vi "内置参数设置.vi"() -> ()   [LabVIEW 2016]
uses:
  <vilib>/Utility/miscctls.llb/LVPointTypeDef.ctl
panel:
  in  "滴定延时时间:\n(单位:毫秒)":u16
  in  "斜率阈值:":dbl
  in  "阀配置:":u8(ring) items=["三通阀", "排阀"]
  in  "AB跨度告警值:":u16
  in  "B值告警上限值:":u16
  in  "B值范围:":u16
  in  "A值告警上限值:":u16
  in  "A值范围:":u16
  in  "是否存在液位检测板:":u16(ring) items=["否", "是"]
  in  "检出限(mg/L):":dbl
  in  "测量精度(mg/L):":dbl
  in  "ILimitDown":dbl
  in  "ILimitUp:":dbl
  in  "K d:":dbl
  in  "K i:":dbl
  in  "K p:":dbl
  in  "加热超时时间:(单位:秒)":dbl
  in  "告警温度:":dbl
  in  "加热温度:  校准参数":dbl
  in  "运行速度:  (修改需要重启)":u16
  in  "偏心轮: 校准参数":dbl
  in  "注射泵加热超时时间(s):":u16
  in  "注射泵保温温度H:":u8
  in  "注射泵\n保温温度L:":u8
  in  "废液通道:":u8
  in  "纯水通道:":u8
  in  "滴定速度:":u16
  in  "出样速度:":u16
  in  "进样速度:":u16
  in  "阀数量:":u8(ring) items=["9通"=9, "12通"=12]
  in  "注射泵型号":u8(ring) items=["TECAN", "润泽", "旋转阀"]
  in  "阈值(高→低)(mg/L):":dbl
  in  "阈值(低→高)(mg/L):":dbl
  in  "检测下限(mg/L):":dbl
  in  "检测上限(mg/L):":dbl
  in  "关闭":bool
  in  "保存":bool
  in  "读取":bool
  # "仪器内部参数设置"
  # "~"
  # "~"
  # "~"
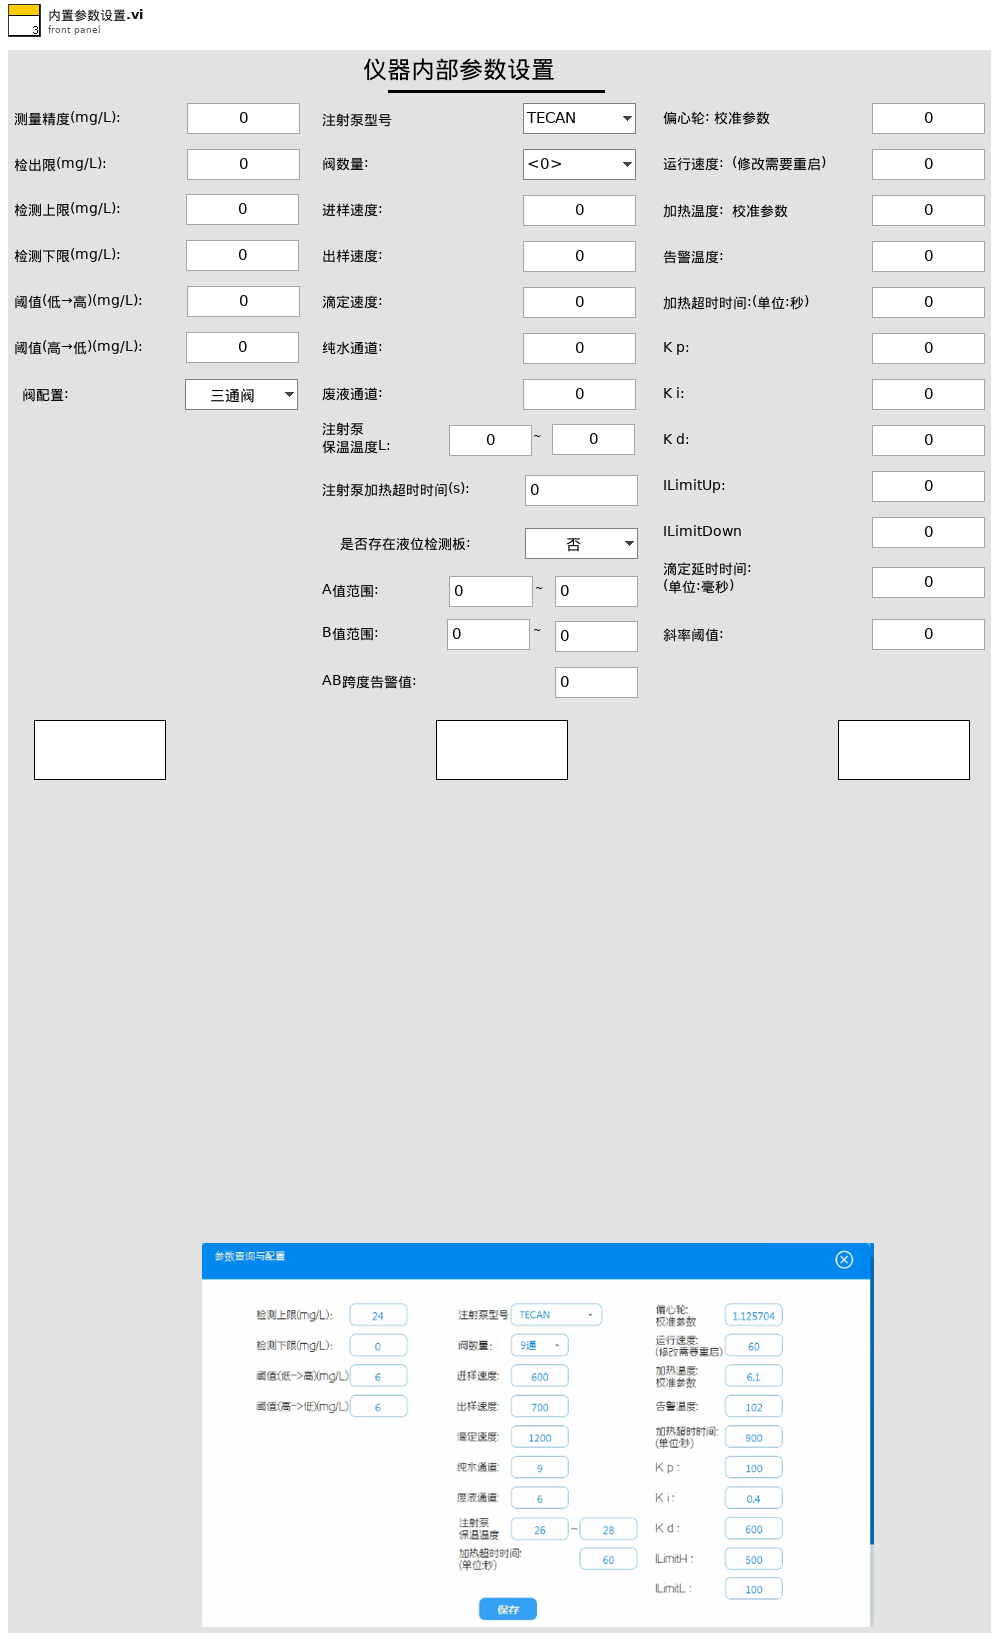
[diagram p1: front panel]
types:
  T1 = typedef "LVPointTypeDef.ctl" = cluster{"Horizontal":i16, "Vertical":i16}
  T2 = cluster{"偏心轮校准参数":dbl, "运行速度(修改需要重启)":u16, "加热温度(校准参数) ":dbl, "告警温度":dbl, "加热超时时间:(单位/秒)":dbl, "K p":dbl, "K i":dbl, "K d":dbl, "ILimitUp":dbl, "ILimitDown":dbl}
  T3 = cluster{"泵类型":u8, "阀数量":u8, "纯水通道":u8, "废液通道":u8, "进样速度":u16, "出样速度":u16, "滴定速度":u16, "注射泵保温温度L":u8, "注射泵保温温度H":u8, "注射泵加热超时时间":u16, "是否存在液位检测板":u16, "A值告警下限值":u16, "A值告警上限值":u16, "B值告警下限值":u16, "B值告警上限值":u16, "AB跨度告警值":u16, "阀配置:":u8, "滴定等待时间":u16, "滴定吸光度斜率":dbl}
  T4 = cluster{"检出限":dbl, "测量精度":dbl, "上限":dbl, "下限":dbl, "阈值（低->高）":dbl, "阈值（高->低）":dbl}
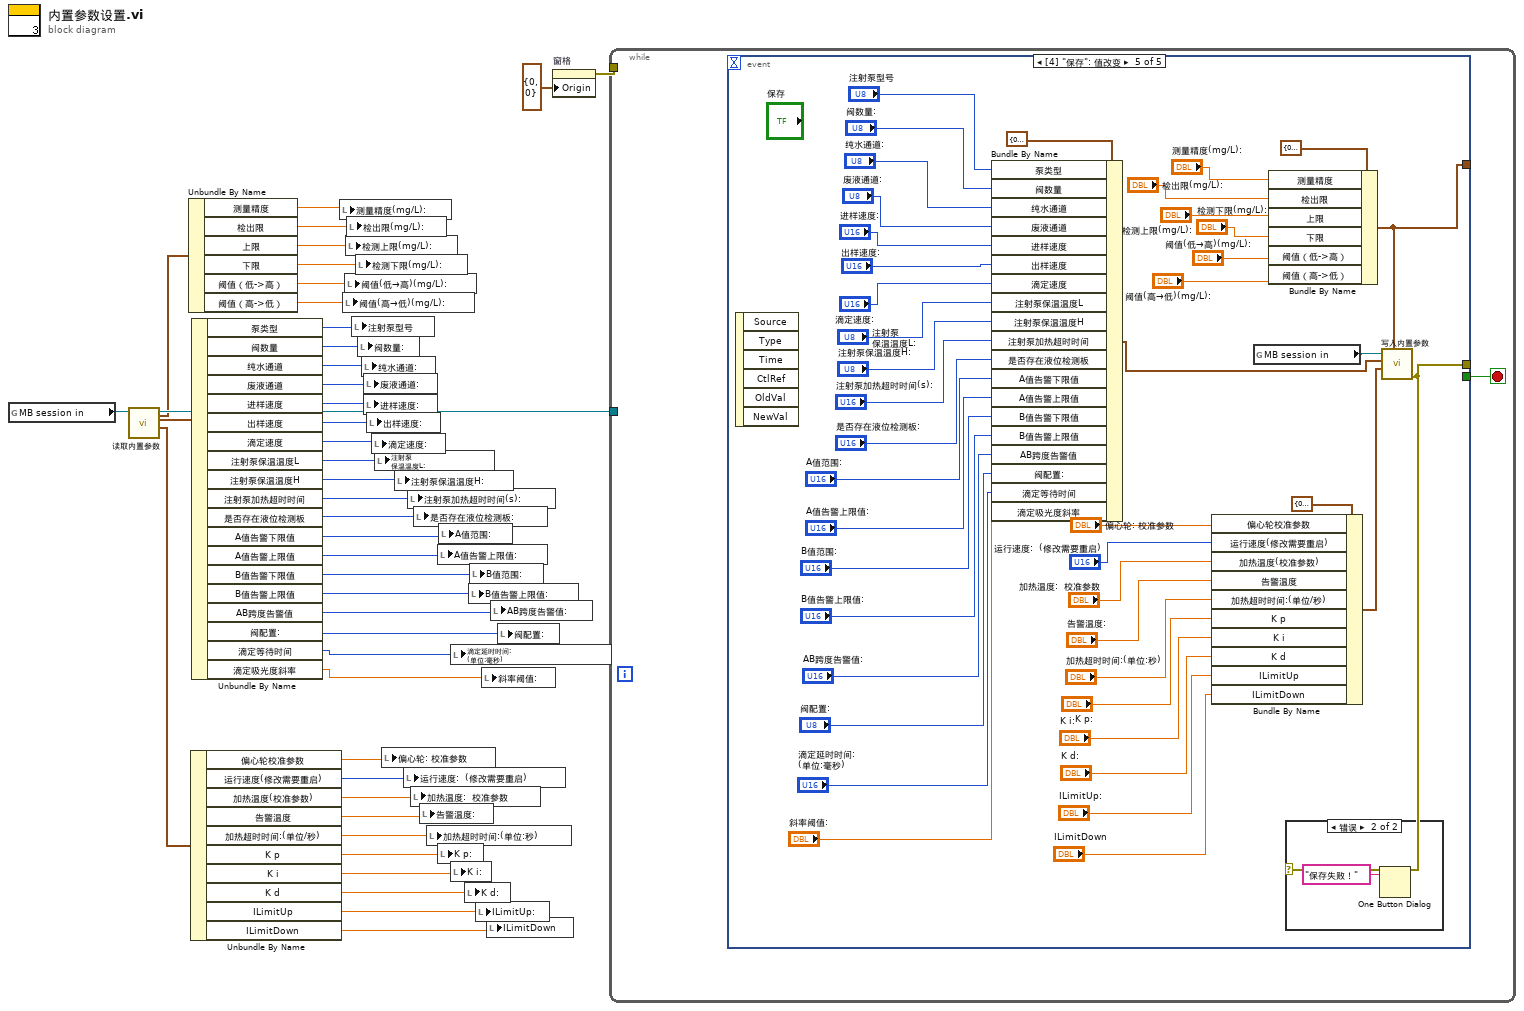
[diagram p0: block diagram]
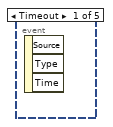
[diagram p2: hidden frame]
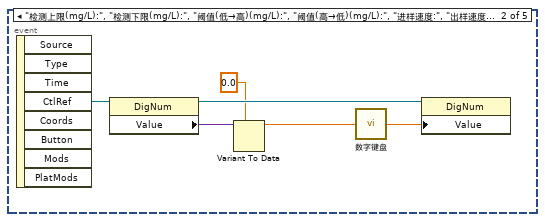
[diagram p3: hidden frame]
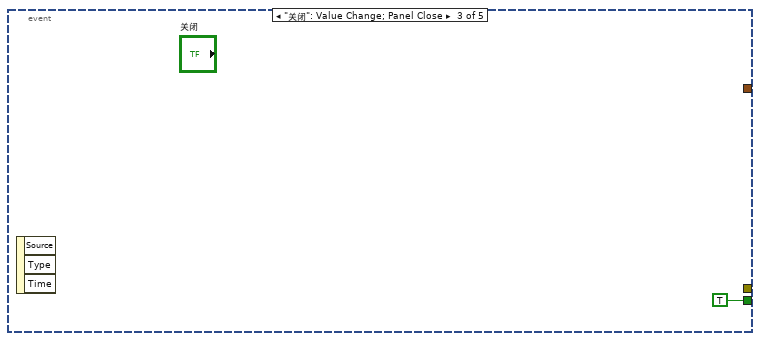
[diagram p4: hidden frame]
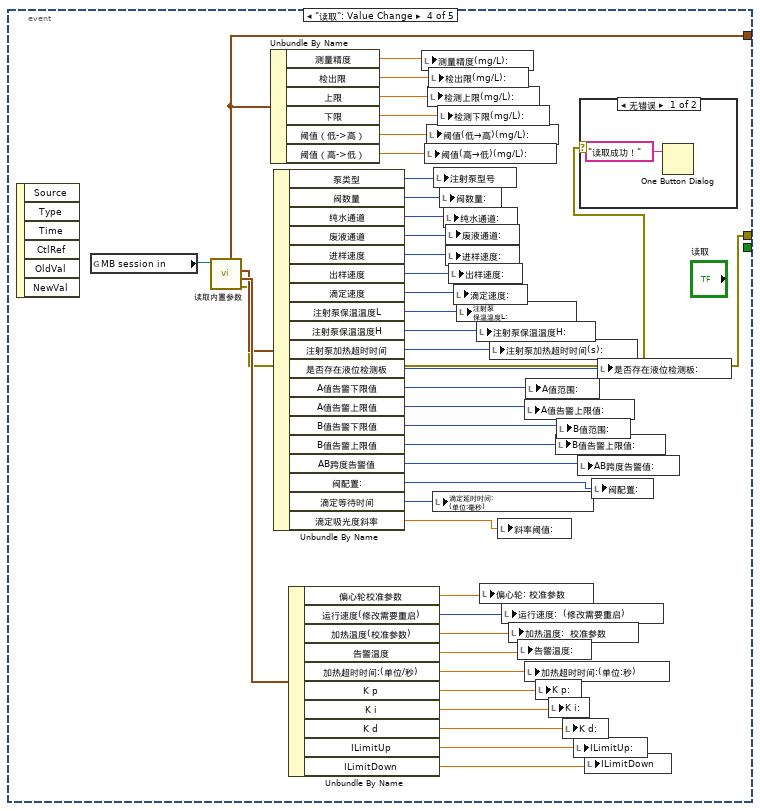
[diagram p5: hidden frame]
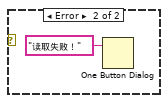
[diagram p6: hidden frame]
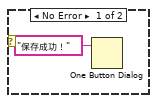
[diagram p7: hidden frame]
diagram:
  n1 = global read "VAR挥发酚全局变量.vi" "MB session in"() -> (w40:refnum<class "MB_Master.lvclass">)
  n2 = call "读取内置参数.vi"("MB session in"=w40) -> ("float"=w37:T2, "外设配置"=w38:T3, "MB session out"=w39:refnum<class "MB_Master.lvclass">, "量程参数读取"=w3:T4)  [unwired: 6 in, 1 out]
  n3 = Unbundle By Name(w3) -> ("测量精度"=w36:dbl, "检出限"=w35:dbl, "上限"=w34:dbl, "下限"=w33:dbl, "阈值（低->高）"=w32:dbl, "阈值（高->低）"=w31:dbl)
  n4 = Unbundle By Name(w37) -> ("偏心轮校准参数"=w20:dbl, "运行速度(修改需要重启)"=w19:u16, "加热温度(校准参数)"=w18:dbl, "告警温度"=w17:dbl, "加热超时时间:(单位/秒)"=w16:dbl, "K p"=w15:dbl, "K i"=w14:dbl, "K d"=w13:dbl, "ILimitUp"=w12:dbl, "ILimitDown"=w11:dbl)
  n5 = Unbundle By Name(w38) -> ("泵类型"=w30:u8, "阀数量"=w29:u8, "纯水通道"=w28:u8, "废液通道"=w27:u8, "进样速度"=w26:u16, "出样速度"=w25:u16, "滴定速度"=w24:u16, "注射泵保温温度L"=w23:u8, "注射泵保温温度H"=w22:u8, "注射泵加热超时时间"=w21:u16, "是否存在液位检测板"=w10:u16, "A值告警下限值"=w9:u16, "A值告警上限值"=w8:u16, "B值告警下限值"=w7:u16, "B值告警上限值"=w6:u16, "AB跨度告警值"=w5:u16, "阀配置:"=w4:u8, "滴定等待时间"=w1:u16, "滴定吸光度斜率"=w2:dbl)
  n6 = local write "测量精度(mg/L):"(w36) -> ()
  n7 = local write "阈值(高→低)(mg/L):"(w31) -> ()
  n8 = local write "阈值(低→高)(mg/L):"(w32) -> ()
  n9 = local write "检测上限(mg/L):"(w34) -> ()
  n10 = local write "检出限(mg/L):"(w35) -> ()
  n11 = local write "注射泵型号"(w30) -> ()
  n12 = local write "检测下限(mg/L):"(w33) -> ()
  n13 = local write "阀数量:"(w29) -> ()
  n14 = local write "纯水通道:"(w28) -> ()
  n15 = local write "废液通道:"(w27) -> ()
  n16 = local write "进样速度:"(w26) -> ()
  n17 = local write "出样速度:"(w25) -> ()
  n18 = local write "滴定速度:"(w24) -> ()
  n19 = local write "注射泵\n保温温度L:"(w23) -> ()
  n20 = local write "偏心轮: 校准参数"(w20) -> ()
  n21 = local write "注射泵保温温度H:"(w22) -> ()
  n22 = local write "运行速度:  (修改需要重启)"(w19) -> ()
  n23 = local write "注射泵加热超时时间(s):"(w21) -> ()
  n24 = local write "加热温度:  校准参数"(w18) -> ()
  n25 = local write "是否存在液位检测板:"(w10) -> ()
  n26 = local write "告警温度:"(w17) -> ()
  n27 = local write "加热超时时间:(单位:秒)"(w16) -> ()
  n28 = local write "A值告警上限值:"(w8) -> ()
  n29 = local write "K p:"(w15) -> ()
  n30 = local write "A值范围:"(w9) -> ()
  n31 = local write "滴定延时时间:\n(单位:毫秒)"(w1) -> ()
  n32 = local write "K i:"(w14) -> ()
  n33 = local write "K d:"(w13) -> ()
  n34 = local write "B值告警上限值:"(w6) -> ()
  n35 = local write "B值范围:"(w7) -> ()
  n36 = local write "ILimitUp:"(w12) -> ()
  n37 = local write "斜率阈值:"(w2) -> ()
  n38 = local write "ILimitDown"(w11) -> ()
  n39 = local write "AB跨度告警值:"(w5) -> ()
  n40 = local write "阀配置:"(w4) -> ()
  n41 = property on="窗格" class="Pane"("Origin"=T1 {"Horizontal"=0, "Vertical"=0} ("原点")) -> (error out=w41:errorcluster)  [unwired: 2 in, 1 out]
  n42 = while {
    tunnel: w41 -> [_]
    tunnel: w39 -> [_]
    stop <- w43 stop-if-true
    n43 = event shown="[4] \"保存\": 值改变" {
      selector: _ -> [_ _ _ _ _]
      dyn-events: _ -> [_ _ _ _ _]
      timeout: _ -> [_ _ _ _ _]
      tunnel: [_ _ TRUE _ _] -> w43
      tunnel: [_ _ _ w61 w106] -> _
      tunnel: [_ _ _ w53 w97] -> _
      event Timeout {
        n44 = event-data() -> ()  [unwired: 1 in, 3 out]
      }
      event "检测上限(mg/L):", "检测下限(mg/L):", "阈值(低→高)(mg/L):", "阈值(高→低)(mg/L):", "进样速度:", "出样速度:", "滴定速度:", "纯水通道:", "废液通道:", "注射泵\n保温温度L:", "注射泵保温温度H:", "注射泵加热超时时间(s):", "偏心轮: 校准参数", "运行速度:  (修改需要重启)", "告警温度:", "加热温度:  校准参数", "K p:", "K i:", "K d:", "ILimitUp:", "ILimitDown", "测量精度(mg/L):", "检出限(mg/L):", "A值范围:", "A值告警上限值:", "B值范围:", "B值告警上限值:", "AB跨度告警值:", "斜率阈值:", "滴定延时时间:\n(单位:毫秒)": Mouse Down {
        n45 = event-data() -> ("CtlRef"=w49:refnum<vi>)  [unwired: 1 in, 7 out]
        n46 = property class="DigNum"(reference=w49) -> (reference out=w48:refnum<vi>, "Value"=w46:variant)  [unwired: 1 in, 1 out]
        n47 = Variant To Data(type=0.0 ("OldNumber"), Variant=w46) -> (data=w44:dbl)  [unwired: 1 in, 1 out]
        n48 = call "数字键盘.vi"("OldNumber"=w44) -> ("NewNumber"=w47:dbl)
        n49 = property class="DigNum"(reference=w48, "Value"=w47) -> ()  [unwired: 1 in, 2 out]
      }
      event "关闭": Value Change; Panel Close {
        n50 = event-data() -> ()  [unwired: 1 in, 3 out]
      }
      event "读取": Value Change {
        n51 = event-data() -> ()  [unwired: 1 in, 6 out]
        n52 = global read "VAR挥发酚全局变量.vi" "MB session in"() -> (w62:refnum<class "MB_Master.lvclass">)
        n53 = call "读取内置参数.vi"("MB session in"=w62) -> ("error out"=w61:errorcluster, "float"=w64:T2, "外设配置"=w63:T3, "量程参数读取"=w53:T4)  [unwired: 6 in, 1 out]
        n54 = Unbundle By Name(w53) -> ("测量精度"=w65:dbl, "检出限"=w66:dbl, "上限"=w67:dbl, "下限"=w68:dbl, "阈值（低->高）"=w69:dbl, "阈值（高->低）"=w70:dbl)
        n55 = Unbundle By Name(w63) -> ("泵类型"=w71:u8, "阀数量"=w72:u8, "纯水通道"=w73:u8, "废液通道"=w74:u8, "进样速度"=w75:u16, "出样速度"=w76:u16, "滴定速度"=w77:u16, "注射泵保温温度L"=w78:u8, "注射泵保温温度H"=w79:u8, "注射泵加热超时时间"=w80:u16, "是否存在液位检测板"=w60:u16, "A值告警下限值"=w59:u16, "A值告警上限值"=w58:u16, "B值告警下限值"=w57:u16, "B值告警上限值"=w56:u16, "AB跨度告警值"=w55:u16, "阀配置:"=w54:u8, "滴定等待时间"=w52:u16, "滴定吸光度斜率"=w51:dbl)
        n56 = Unbundle By Name(w64) -> ("偏心轮校准参数"=w81:dbl, "运行速度(修改需要重启)"=w82:u16, "加热温度(校准参数)"=w83:dbl, "告警温度"=w84:dbl, "加热超时时间:(单位/秒)"=w85:dbl, "K p"=w86:dbl, "K i"=w87:dbl, "K d"=w88:dbl, "ILimitUp"=w89:dbl, "ILimitDown"=w90:dbl)
        n57 = local write "测量精度(mg/L):"(w65) -> ()
        n58 = local write "阈值(高→低)(mg/L):"(w70) -> ()
        n59 = local write "阈值(低→高)(mg/L):"(w69) -> ()
        n60 = local write "检测上限(mg/L):"(w67) -> ()
        n61 = local write "检出限(mg/L):"(w66) -> ()
        n62 = local write "滴定延时时间:\n(单位:毫秒)"(w52) -> ()
        n63 = local write "注射泵型号"(w71) -> ()
        n64 = local write "检测下限(mg/L):"(w68) -> ()
        n65 = local write "阀数量:"(w72) -> ()
        n66 = local write "纯水通道:"(w73) -> ()
        n67 = local write "废液通道:"(w74) -> ()
        n68 = local write "进样速度:"(w75) -> ()
        n69 = local write "出样速度:"(w76) -> ()
        n70 = local write "滴定速度:"(w77) -> ()
        n71 = local write "注射泵\n保温温度L:"(w78) -> ()
        n72 = local write "注射泵保温温度H:"(w79) -> ()
        n73 = local write "偏心轮: 校准参数"(w81) -> ()
        n74 = local write "注射泵加热超时时间(s):"(w80) -> ()
        n75 = local write "斜率阈值:"(w51) -> ()
        n76 = local write "运行速度:  (修改需要重启)"(w82) -> ()
        n77 = local write "加热温度:  校准参数"(w83) -> ()
        n78 = local write "告警温度:"(w84) -> ()
        n79 = local write "A值告警上限值:"(w58) -> ()
        n80 = local write "加热超时时间:(单位:秒)"(w85) -> ()
        n81 = local write "A值范围:"(w59) -> ()
        n82 = local write "K p:"(w86) -> ()
        n83 = local write "K i:"(w87) -> ()
        n84 = local write "B值告警上限值:"(w56) -> ()
        n85 = local write "B值范围:"(w57) -> ()
        n86 = local write "K d:"(w88) -> ()
        n87 = local write "ILimitUp:"(w89) -> ()
        n88 = local write "AB跨度告警值:"(w55) -> ()
        n89 = case shown="无错误" w61 {
          frame No Error {
            n90 = One Button Dialog(message="读取成功！" ("消息")) -> ()  [unwired: 1 in, 1 out]
          }
          frame Error {
            n91 = One Button Dialog(message="读取失败！" ("消息")) -> ()  [unwired: 1 in, 1 out]
          }
        }
        n92 = local write "ILimitDown"(w90) -> ()
        n93 = local write "阀配置:"(w54) -> ()
        n94 = local write "是否存在液位检测板:"(w60) -> ()
      }
      event "保存": Value Change {
        n95 = event-data() -> ()  [unwired: 1 in, 6 out]
        n96 = Bundle By Name(cluster=T3 {"泵类型"=0, "阀数量"=0, "纯水通道"=0, "废液通道"=0, "进样速度"=0, "出样速度"=0, "滴定速度"=0, "注射泵保温温度L"=0, "注射泵保温温度H"=0, "注射泵加热超时时间"=0, "是否存在液位检测板"=0, "A值告警下限值"=0, "A值告警上限值"=0, "B值告警下限值"=0, "B值告警上限值"=0, "AB跨度告警值"=0, "阀配置:"=0, "滴定等待时间"=0, "滴定吸光度斜率"=0.0} ("外设配置"), "泵类型"="注射泵型号", "阀数量"="阀数量:", "纯水通道"="纯水通道:", "废液通道"="废液通道:", "进样速度"="进样速度:", "出样速度"="出样速度:", "滴定速度"="滴定速度:", "注射泵保温温度L"="注射泵\n保温温度L:", "注射泵保温温度H"="注射泵保温温度H:", "注射泵加热超时时间"="注射泵加热超时时间(s):", "是否存在液位检测板"="是否存在液位检测板:", "A值告警下限值"="A值范围:", "A值告警上限值"="A值告警上限值:", "B值告警下限值"="B值范围:", "B值告警上限值"="B值告警上限值:", "AB跨度告警值"="AB跨度告警值:", "阀配置:"="阀配置:", "滴定等待时间"="滴定延时时间:\n(单位:毫秒)", "滴定吸光度斜率"="斜率阈值:") -> (w94:T3)
        n97 = Bundle By Name(cluster=T2 {"偏心轮校准参数"=0.0, "运行速度(修改需要重启)"=0, "加热温度(校准参数) "=0.0, "告警温度"=0.0, "加热超时时间:(单位/秒)"=0.0, "K p"=0.0, "K i"=0.0, "K d"=0.0, "ILimitUp"=0.0, "ILimitDown"=0.0} ("float"), "偏心轮校准参数"="偏心轮: 校准参数", "运行速度(修改需要重启)"="运行速度:  (修改需要重启)", "加热温度(校准参数)"="加热温度:  校准参数", "告警温度"="告警温度:", "加热超时时间:(单位/秒)"="加热超时时间:(单位:秒)", "K p"="K p:", "K i"="K i:", "K d"="K d:", "ILimitUp"="ILimitUp:", "ILimitDown"="ILimitDown") -> (w107:T2)
        n98 = global read "VAR挥发酚全局变量.vi" "MB session in"() -> (w135:refnum<class "MB_Master.lvclass">)
        n99 = Bundle By Name(cluster=T4 {"检出限"=0.0, "测量精度"=0.0, "上限"=0.0, "下限"=0.0, "阈值（低->高）"=0.0, "阈值（高->低）"=0.0} ("量程参数读取"), "测量精度"="测量精度(mg/L):", "检出限"="检出限(mg/L):", "上限"="检测上限(mg/L):", "下限"="检测下限(mg/L):", "阈值（低->高）"="阈值(低→高)(mg/L):", "阈值（高->低）"="阈值(高→低)(mg/L):") -> (w97:T4)
        n100 = call "写入内置参数.vi"("量程参数读取"=w97, "float"=w107, "外设配置"=w94, "MB session in"=w135) -> ("error out"=w106:errorcluster)  [unwired: 6 in, 1 out]
        n101 = case shown="错误" w106 {
          frame No Error {
            n102 = One Button Dialog(message="保存成功！" ("消息")) -> ()  [unwired: 1 in, 1 out]
          }
          frame Error {
            n103 = One Button Dialog(message="保存失败！" ("消息")) -> ()  [unwired: 1 in, 1 out]
          }
        }
      }
    }
  }
